vi "seleccionarTableName.vi"(11 "datosClaseDB in":T1) -> (3 "tableNameOut":string)   [LabVIEW 2014]
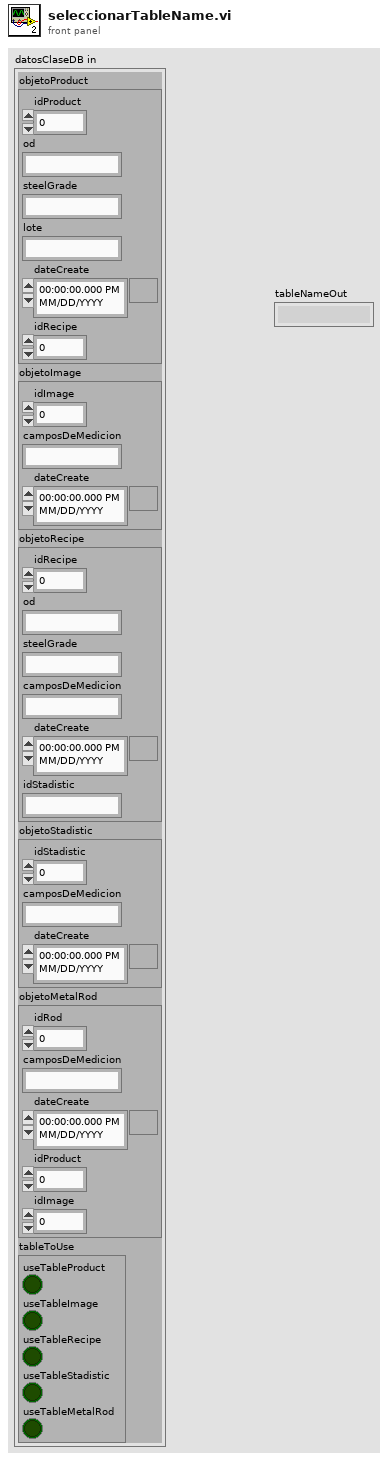
[diagram p1: front panel]
types:
  T1 = cluster{"objetoProduct":cluster{"idProduct":dbl, "od":string, "steelGrade":string, "lote":string, "dateCreate":timestamp, "idRecipe":dbl}, "objetoImage":cluster{"idImage":dbl, "camposDeMedicion":string, "dateCreate":timestamp}, "objetoRecipe":cluster{"idRecipe":dbl, "od":string, "steelGrade":string, "camposDeMedicion":string, "dateCreate":timestamp, "idStadistic":string}, "objetoStadistic":cluster{"idStadistic":dbl, "camposDeMedicion":string, "dateCreate":timestamp}, "objetoMetalRod":cluster{"idRod":dbl, "camposDeMedicion":string, "dateCreate":timestamp, "idProduct":dbl, "idImage":dbl}, "tableToUse":cluster{"useTableProduct":bool, "useTableImage":bool, "useTableRecipe":bool, "useTableStadistic":bool, "useTableMetalRod":bool}}
  T2 = cluster{"useTableProduct":bool, "useTableImage":bool, "useTableRecipe":bool, "useTableStadistic":bool, "useTableMetalRod":bool}
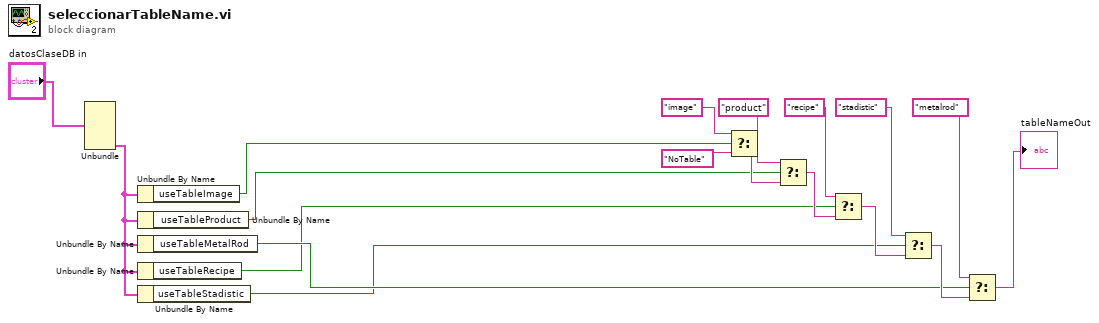
[diagram p0: block diagram]
diagram:
  n1 = Unbundle("datosClaseDB in") -> ("tableToUse"=w7:T2)  [unwired: 5 out]
  n2 = Unbundle By Name(w7) -> ("useTableImage"=w5:bool)
  n3 = Unbundle By Name(w7) -> ("useTableProduct"=w4:bool)
  n4 = Unbundle By Name(w7) -> ("useTableMetalRod"=w3:bool)
  n5 = Unbundle By Name(w7) -> ("useTableRecipe"=w2:bool)
  n6 = Unbundle By Name(w7) -> ("useTableStadistic"=w1:bool)
  n7 = Select(t="image", s=w5, f="NoTable") -> (s? t:f=w17:string)
  n8 = Select(t="product", s=w4, f=w17) -> (s? t:f=w15:string)
  n9 = Select(t="recipe", s=w2, f=w15) -> (s? t:f=w13:string)
  n10 = Select(t="stadistic", s=w1, f=w13) -> (s? t:f=w11:string)
  n11 = Select(t="metalrod", s=w3, f=w11) -> (s? t:f=→"tableNameOut":string)
